vi "Get Users With Attribute Name.vi"(0 "User Configuration Manager in":refnum<class "User Configuration Manager.lvclass">, 5 "Attribute Name":string, 11 "error in (no error)":errorcluster) -> (4 "User Configuration Manager out":refnum<class "User Configuration Manager.lvclass">, 6 "Users":string[](array[string]), 8 "Number of Users Found":u32, 15 "error out":errorcluster)   [LabVIEW 2020, in "User Configuration Manager.lvlib" / "User Configuration Manager.lvclass"]
doc: "Returns all users with the an attribute named Attribute Name."
uses:
  <vilib>/gpm_packages/@cs/user-manager/Source/User Configuration Manager/User Configuration Manager.lvclass
  <vilib>/gpm_packages/@cs/user-manager/Source/User Configuration Manager/User Configuration Manager.lvclass/User Configuration Manager.ctl
  1eee3069-f19d-4a03-a5c3-f2487ffa0efd.vi
  <vilib>/gpm_packages/@cs/user-manager/Source/User Configuration Manager/Accessors/Read Linked List Ref .vi
  <vilib>/gpm_packages/@cs/linked-list/Source/Linked List/ILinkedList/ILinked List.lvclass
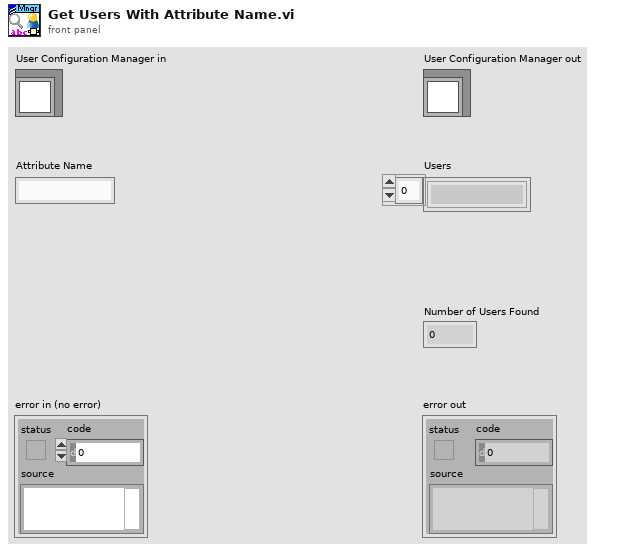
[diagram p1: front panel]
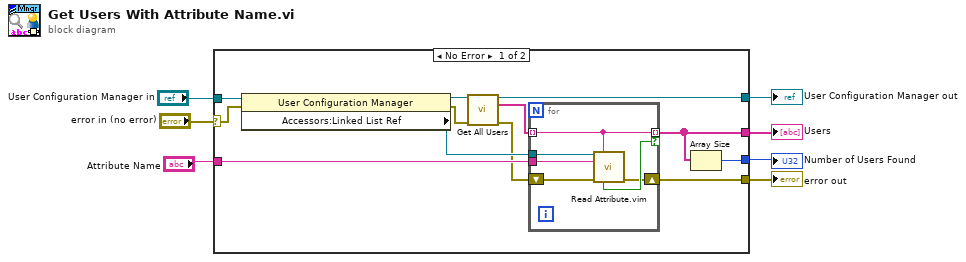
[diagram p0: block diagram]
diagram:
  n1 = case shown="No Error" "error in (no error)" {
    selector: "error in (no error)" -> [w18 w27]
    tunnel: "User Configuration Manager in" -> [w19 w26]
    tunnel: [w9 w26] -> w5
    tunnel: [w13 w27] -> w4
    tunnel: "Attribute Name" -> [w15 _]
    tunnel: [w17 _] -> w2
    tunnel: [w14 _] -> w1
    frame No Error {
      n2 = property class="User Configuration Manager"(reference=w19, error in=w18) -> (reference out=w12:refnum<class "User Configuration Manager.lvclass">, error out=w11:errorcluster, "Accessors:Linked List Ref "=w16:refnum<data-value>)
      n3 = call-dynamic "Get All Users.vi"("User Configuration Manager in"=w12, "error in (no error)"=w11) -> ("User Configuration Manager out"=w9:refnum<class "User Configuration Manager.lvclass">, "Users"=w8:string[], "error out"=w10:errorcluster)  [unwired: 10 in, 1 out]
      n4 = for {
        tunnel: w16 -> [w25]
        tunnel: w8 -> [w23] mode=indexing
        tunnel: w15 -> [w24]
        tunnel: [w23] -> w14 mode=indexing if=w22
        shift-right: [w20] -> w13
        shift-left: w10 -> [w21]
        n5 = call "Read Attribute.vim"("Linked List Ref"=w25, "Linked List ID"=w23, "Attribute Name"=w24, "error in (no error)"=w21) -> ("Found?"=w22:bool, "error out"=w20:errorcluster)  [unwired: 6 in, 4 out]
      }
      n6 = Array Size(array=w14) -> (size(s)=w17:i32)
    }
    frame Error {
    }
  }
  "error out" <- w4
  "User Configuration Manager out" <- w5
  "Users" <- w1
  "Number of Users Found" <- w2
